vi "AlazarWriteRegister.vi"(0 "Board Handle":u64, 5 "Offset":u32, 7 "Value":u32, 9 "Password":u32, 11 "error in (no error)":errorcluster) -> (4 "Board Handle Out":u64, 10 "Return Code":u32, 15 "error out":errorcluster)   [LabVIEW 2009]
uses:
  ATSApi.dll
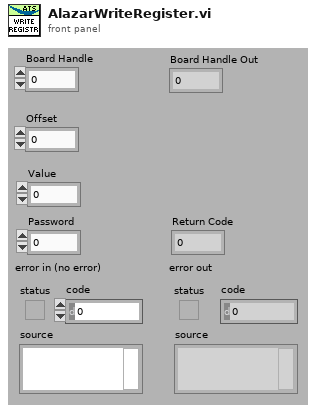
[diagram p1: front panel]
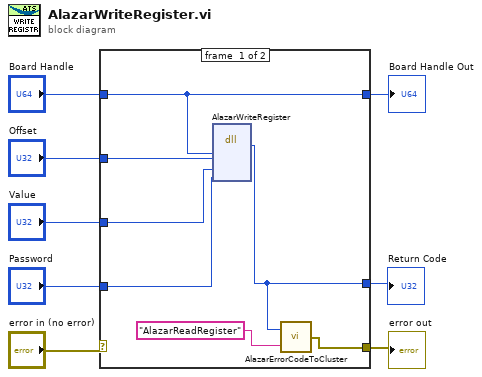
[diagram p0: block diagram]
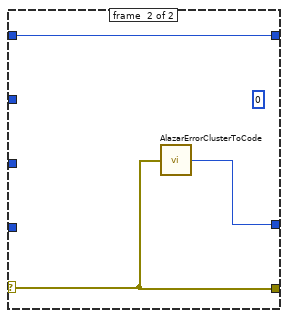
[diagram p2: hidden frame]
diagram:
  n1 = case shown="No Error" "error in (no error)" {
    selector: "error in (no error)" -> [_ w17]
    tunnel: [w10 w17] -> w7
    tunnel: [w15 w18] -> w6
    tunnel: "Board Handle" -> [w15 w18]
    tunnel: [w12 w16] -> w4
    tunnel: "Offset" -> [w14 _]
    tunnel: "Password" -> [w13 _]
    tunnel: "Value" -> [w9 _]
    frame #0 {
      n2 = dll-call lib="ATSApi.dll" fn="AlazarWriteRegister"("handle"=w15, "offset"=w14, "val"=w9, "password"=w13) -> ("return type"=w12:u32)  [unwired: 7 in, 2 out]
      n3 = call "AlazarErrorCodeToCluster.vi"("Message"="AlazarReadRegister", "Error Code"=w12) -> ("error out"=w10:errorcluster)
    }
    frame #1 {
      (unwired) u32 0
      n4 = call "AlazarErrorClusterToCode.vi"("error in (no error)"=w17) -> ("Error Code"=w16:u32)
    }
  }
  "Board Handle Out" <- w6
  "error out" <- w7
  "Return Code" <- w4
